vi "Cron Basic Job Execution.vi"() -> ()   [LabVIEW 2013]
uses:
  Job/Job Report -- cluster.ctl
  Job/Job.lvclass/Job.ctl
  JobReport/JobReport.lvclass/JobReport.ctl
  Cron/Create Cron Expression.vi
  Cron/Compute Next Cron.vi
  Cron.Quartz/Cron.Quartz.lvclass
  openCron.lvlib
  Job/Job.lvclass
  Job.StaticVIRef/Job.StaticVIRef.lvclass
  JobReport/JobReport.lvclass
panel:
  out "Map":variant
  out "last error":errorcluster
  out "syntax valid?":bool
  in  "Cron Expression":string="0/10 * * ? * *"
  out "Job Report":T1
  in  "Kill Job":bool
  in  "Abort Job":bool
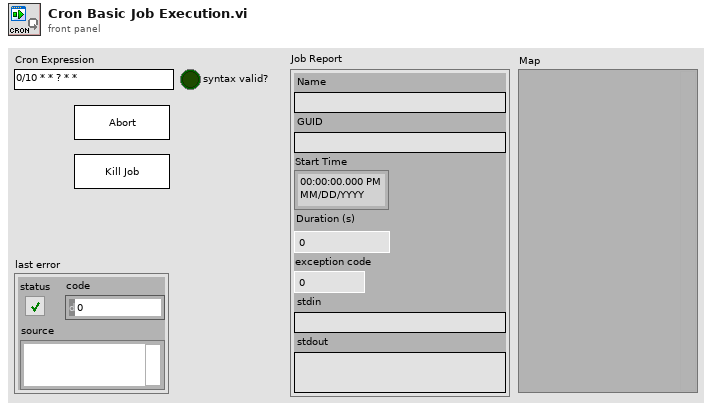
[diagram p1: front panel]
types:
  T1 = typedef "openCronJob.lvlib/JobReport.lvclass/Job Report -- cluster.ctl" = cluster{"Name":string, "GUID":string, "Start Time":timestamp, "Duration (s)":dbl, "exception code":i32, "stdin":string, "stdout":string}
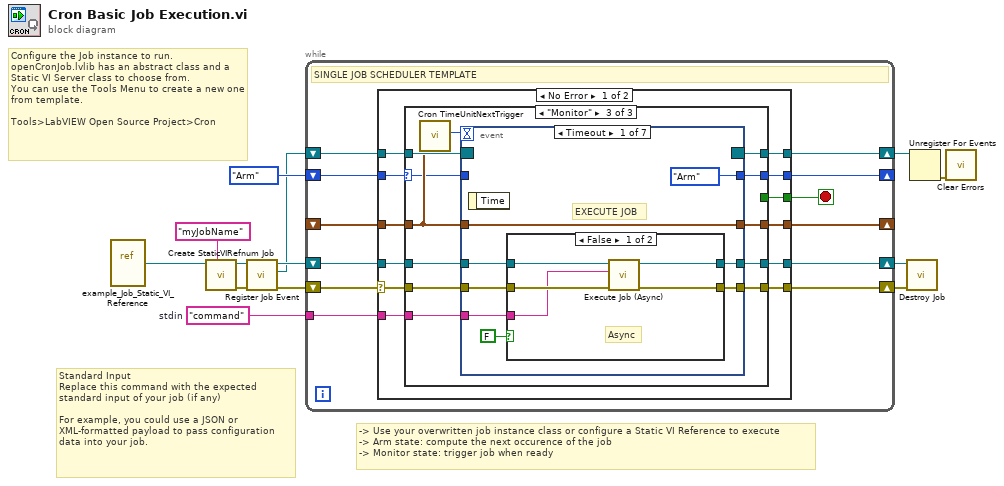
[diagram p0: block diagram]
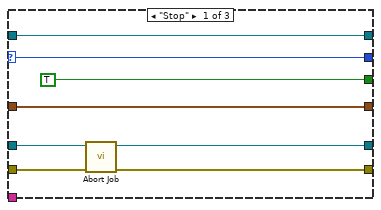
[diagram p2: hidden frame]
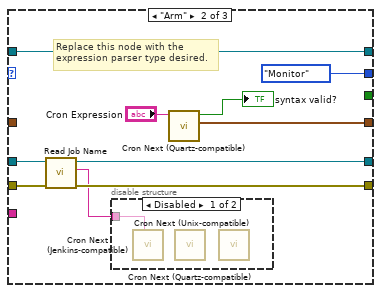
[diagram p3: hidden frame]
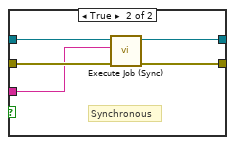
[diagram p5: hidden frame]
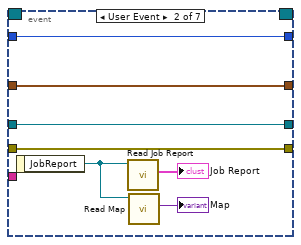
[diagram p6: hidden frame]
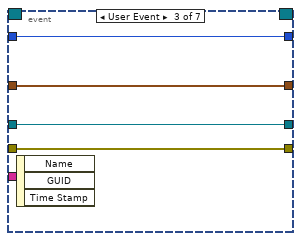
[diagram p7: hidden frame]
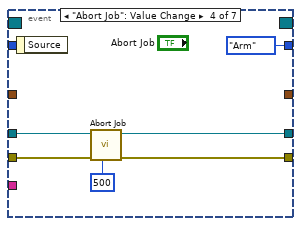
[diagram p8: hidden frame]
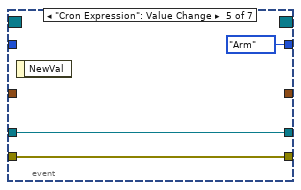
[diagram p9: hidden frame]
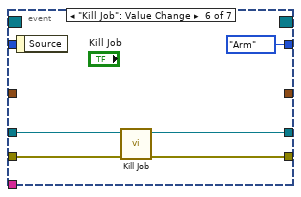
[diagram p10: hidden frame]
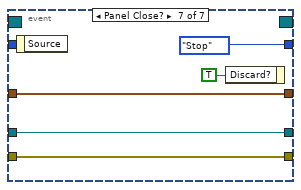
[diagram p11: hidden frame]
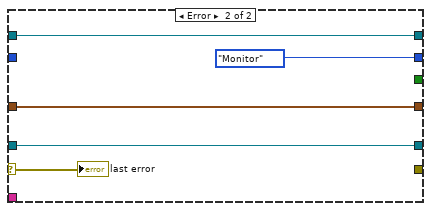
[diagram p12: hidden frame]
diagram:
  w1 = "command"  # stdin
  # "Standard Input\nReplace this command with the expected standard input of your job (if any)\n\nFor example, you could use a JSON or XML-formatted payload to pass configuration data into your job."
  # "Configure the Job instance to run.\nopenCronJob.lvlib has an abstract class and a Static VI Server class to choose from.\nYou can use the Tools Menu to create a new one from template.\n\nTools>LabVIEW Open Source Project>Cron"
  # "-> Use your overwritten job instance class or configure a Static VI Reference to execute\n-> Arm state: compute the next occurence of the job\n-> Monitor state: trigger job when ready"
  n1 = vi-ref "example_Job_Static_VI_Reference.vi"() -> (w2:refnum<vi>)
  n2 = call "Create StaticVIRefnum Job.vi"("Job Name"="myJobName", "Static VI Refnum"=w2) -> ("error out"=w6:errorcluster, "Job.StaticVIRef out"=w8:refnum<class "Job.StaticVIRef.lvclass">)  [unwired: 8 in]
  n3 = call "Register Job Event.vi"("Job in"=w8) -> ("Job Event Registration"=w4:refnum<event-registration>, "Job out"=w7:refnum<class "Job.StaticVIRef.lvclass">)  [unwired: 9 in]
  n4 = while {
    shift-right: [w23] -> _
    shift-left: _ -> [w24]
    shift-right: [w21] -> _
    shift-left: enum16{"Arm", "Stop", "Monitor"}."Arm" -> [w22]
    shift-right: [w18] -> w11
    shift-left: w4 -> [w19]
    shift-right: [w16] -> w9
    shift-left: w7 -> [w17]
    shift-right: [w15] -> w5
    shift-left: w6 -> [w14]
    tunnel: w1 -> [w13]
    stop <- w20 stop-if-true
    # "SINGLE JOB SCHEDULER TEMPLATE"
    n5 = case shown="No Error" w14 {
      selector: w14 -> [w26 w116]
      tunnel: w24 -> [w36 w118]
      tunnel: [w35 w118] -> w23
      tunnel: w22 -> [w34 _]
      tunnel: [w33 enum16{"Arm", "Stop", "Monitor"}."Monitor"] -> w21
      tunnel: [w32 _] -> w20
      tunnel: w19 -> [w31 w120]
      tunnel: [w30 w120] -> w18
      tunnel: w17 -> [w29 w117]
      tunnel: [w28 w117] -> w16
      tunnel: [w27 _] -> w15
      tunnel: w13 -> [w25 _]
      frame No Error {
        n6 = case shown="\"Monitor\"" w34 {
          selector: w34 -> [w44 _ w59]
          tunnel: w36 -> [w42 _ w62]
          tunnel: [w42 w53 w64] -> w35
          tunnel: [w44 enum16{"Arm", "Stop", "Monitor"}."Monitor" w65] -> w33
          tunnel: [TRUE _ _] -> w32
          tunnel: w31 -> [w41 w54 w67]
          tunnel: [w41 w54 w66] -> w30
          tunnel: w29 -> [w40 w47 w61]
          tunnel: [w39 w46 w60] -> w28
          tunnel: w26 -> [w38 w49 w58]
          tunnel: [w37 w48 w57] -> w27
          tunnel: w25 -> [_ _ w56]
          frame "Stop" {
            n7 = call "Abort Job.vi"("error in (no error)"=w38, "Job in"=w40) -> ("error out"=w37:errorcluster, "Job out"=w39:refnum<class "Job.StaticVIRef.lvclass">)  [unwired: 5 in, 3 out]
          }
          frame "Arm" {
            # "Replace this node with the\nexpression parser type desired."
            n8 = call "Read Job Name.vi"("error in (no error)"=w49, "Job in"=w47) -> ("error out"=w48:errorcluster, "Name"=w45:string, "Job out"=w46:refnum<class "Job.StaticVIRef.lvclass">)  [unwired: 7 in]
            n9 = disable-structure shown="Disabled" {
              disable-tunnel: w45 -> [w55 _]
              frame Disabled {
                n10 = call "Cron Next (Jenkins-compatible).vi"("Job Name"=w55) -> ()  [unwired: 8 in, 3 out]
                n11 = call "Cron Next (Quartz-compatible).vi"() -> ()  [unwired: 9 in, 3 out]
                n12 = call "Cron Next (Unix-compatible).vi"() -> ()  [unwired: 9 in, 3 out]
              }
              frame Enabled {
              }
            }
            n13 = call "Cron Next (Quartz-compatible).vi"("Cron Expression"="Cron Expression") -> ("Next Occurence"=w53:timestamp, "syntax valid?"=→"syntax valid?":bool)  [unwired: 8 in, 1 out]
          }
          frame "Monitor" {
            n14 = call "Cron TimeUnitNextTrigger.vi"("Next Occurence"=w62) -> ("next event (ms)"=w63:i32)  [unwired: 10 in]
            n15 = event shown="[0] Timeout" {
              selector: w67 -> [_ _ _ _ _ _ _]
              dyn-events: [_ _ _ _ _ _ _] -> w66
              timeout: w63 -> [_ _ _ _ _ _ _]
              tunnel: [enum16{"Arm", "Stop", "Monitor"}."Arm" w91 w95 enum16{"Arm", "Stop", "Monitor"}."Arm" enum16{"Arm", "Stop", "Monitor"}."Arm" enum16{"Arm", "Stop", "Monitor"}."Arm" enum16{"Arm", "Stop", "Monitor"}."Stop"] -> w65
              tunnel: [w69 w92 w96 _ _ _ w113] -> w64
              tunnel: w62 -> [w69 w92 w96 _ _ _ w113]
              tunnel: w61 -> [w74 w90 w94 w101 w104 w109 w112]
              tunnel: [w72 w90 w94 w100 w104 w108 w112] -> w60
              tunnel: w59 -> [_ w91 w95 _ _ _ _]
              tunnel: w58 -> [w71 w89 w93 w98 w103 w107 w111]
              tunnel: [w70 w89 w93 w97 w103 w106 w111] -> w57
              tunnel: w56 -> [w68 _ _ _ _ _ _]
              event Timeout {
                # "EXECUTE JOB"
                n16 = event-data() -> ()  [unwired: 1 in, 1 out]
                n17 = case shown="False" FALSE ("Synchronous?") {
                  tunnel: w74 -> [w80 w85]
                  tunnel: [w79 w84] -> w72
                  tunnel: w71 -> [w77 w83]
                  tunnel: [w78 w82] -> w70
                  tunnel: w68 -> [w76 w81]
                  frame False {
                    # "Async"
                    n18 = call "Execute Job (Async).vi"("error in (no error)"=w77, "stdin"=w76, "Job in"=w80) -> ("error out"=w78:errorcluster, "Job out"=w79:refnum<class "Job.StaticVIRef.lvclass">)  [unwired: 6 in, 1 out]
                  }
                  frame True {
                    # "Synchronous"
                    n19 = call "Execute Job (Sync).vi"("error in (no error)"=w83, "stdin"=w81, "Job in"=w85) -> ("error out"=w82:errorcluster, "Job out"=w84:refnum<class "Job.StaticVIRef.lvclass">)  [unwired: 5 in, 2 out]
                  }
                }
              }
              event User Event {
                n20 = event-data() -> ("JobReport"=w87:refnum<class "JobReport.lvclass">)  [unwired: 1 in]
                n21 = call "Read Job Report.vi"("JobReport in"=w87) -> ("Job Report"=→"Job Report":T1)  [unwired: 8 in, 2 out]
                n22 = call "Read Map.vi"("JobReport in"=w87) -> ("Map"=→"Map":variant)  [unwired: 8 in, 2 out]
              }
              event User Event {
                n23 = event-data() -> ()  [unwired: 1 in, 3 out]
              }
              event "Abort Job": Value Change {
                n24 = event-data() -> ()  [unwired: 1 in, 1 out]
                n25 = call "Abort Job.vi"("timeout (500 ms)"=500, "error in (no error)"=w98, "Job in"=w101) -> ("error out"=w97:errorcluster, "Job out"=w100:refnum<class "Job.StaticVIRef.lvclass">)  [unwired: 4 in, 3 out]
              }
              event "Cron Expression": Value Change {
                n26 = event-data() -> ()  [unwired: 1 in, 1 out]
              }
              event "Kill Job": Value Change {
                n27 = event-data() -> ()  [unwired: 1 in, 1 out]
                n28 = call "Kill Job.vi"("error in (no error)"=w107, "Job in"=w109) -> ("error out"=w106:errorcluster, "Job out"=w108:refnum<class "Job.StaticVIRef.lvclass">)  [unwired: 8 in]
              }
              event Panel Close? {
                n29 = event-data() -> ()  [unwired: 1 in, 1 out]
                n30 = event-data("Discard?"=TRUE) -> ()  [unwired: 1 in, 1 out]
              }
            }
          }
        }
      }
      frame Error {
        "last error" <- w116
      }
    }
  }
  n31 = call "Destroy Job.vi"("error in (no error)"=w5, "Job in"=w9) -> ()  [unwired: 8 in, 2 out]
  n32 = Unregister For Events(event registration refnum=w11) -> (error out=w10:errorcluster)  [unwired: 1 in]
  n33 = call <vilib>:"Clear Errors.vi"("error in (no error)"=w10) -> ()  [unwired: 6 in, 1 out]
